vi "Create Sequence Parameter Assignment (Imported Double Array).vi"(4 "Import Length (0: import rest)":u64, 6 "Import Offset (0)":u64, 7 "File Path":path, 8 "error in (no error)":errorcluster, 9 "Channel":string, 10 "Channel Group":string, 11 "Parameter Name":string) -> (0 "error out":errorcluster, 3 "Sequence Parameter Assignment Ref":T1)   [LabVIEW 2020, in "NI_VS Sequence Execution Interface.lvlib"]
doc: "Assigns a value to a real-time sequence parameter. The value can be a constant value, data in a file, or a mapping to a channel in a system definition file. Use this VI to create parameter assignment references to use with the Create Sequence Call VI. \n\nWire data to the <B>Channel</B> input to determine the polymorphic instance to use or manually select the instance."
uses:
  <vilib>/NI VeriStand/Execution/SequenceExecutionInterface/NI_VS Sequence Execution Interface.lvlib
  <vilib>/NI VeriStand/Execution/SequenceExecutionInterface/Sequence Input Assignment Ref.ctl
  NationalInstruments.VeriStand.ClientAPI
  NationalInstruments.VeriStand.DataTypes
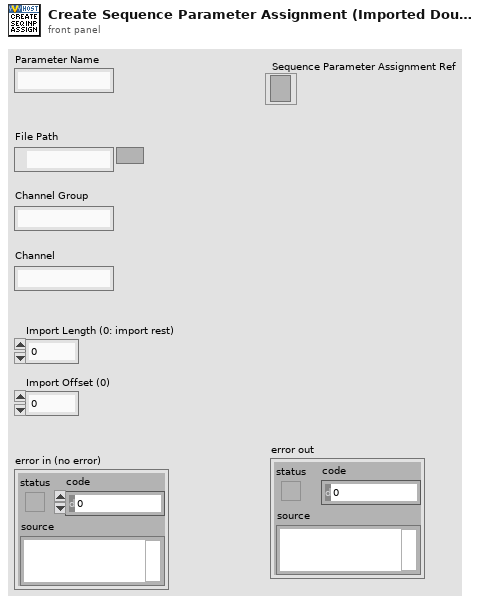
[diagram p1: front panel]
types:
  T1 = typedef "NI_VS Sequence Execution Interface.lvlib/Sequence Input Assignment Ref.ctl" = refnum<k24>
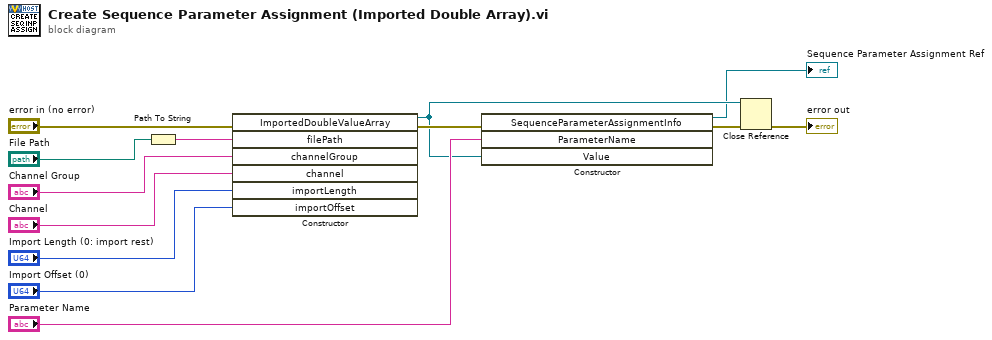
[diagram p0: block diagram]
diagram:
  n1 = Path To String(path="File Path") -> (string=w3:string)
  n2 = constructor class="ImportedDoubleValueArray"(error in="error in (no error)", "filePath"=w3, "channelGroup"="Channel Group", "channel"="Channel", "importLength"="Import Length (0: import rest)", "importOffset"="Import Offset (0)") -> (reference out=w10:refnum<k24>, error out=w13:errorcluster)  [unwired: 2 in, 6 out]
  n3 = constructor class="SequenceParameterAssignmentInfo"(error in=w13, "ParameterName"="Parameter Name", "Value"=w10) -> (reference out=→"Sequence Parameter Assignment Ref":refnum<k24>, error out=w11:errorcluster)  [unwired: 2 in, 3 out]
  n4 = Close Reference(reference=w10, error in (no error)=w11) -> (error out=→"error out":errorcluster)
